vi "Main.vi"() -> ()   [LabVIEW 2016]
uses:
  Globale Variable/Globale Variable.vi
panel:
  in  "LAUNCH":bool
  in  "voltage_start":dbl
  in  "starting threshold":dbl
  in  "v_max":dbl
  in  "k_lqr":dbl
  out "error out":errorcluster
  in  "lambda_target":dbl=0.1
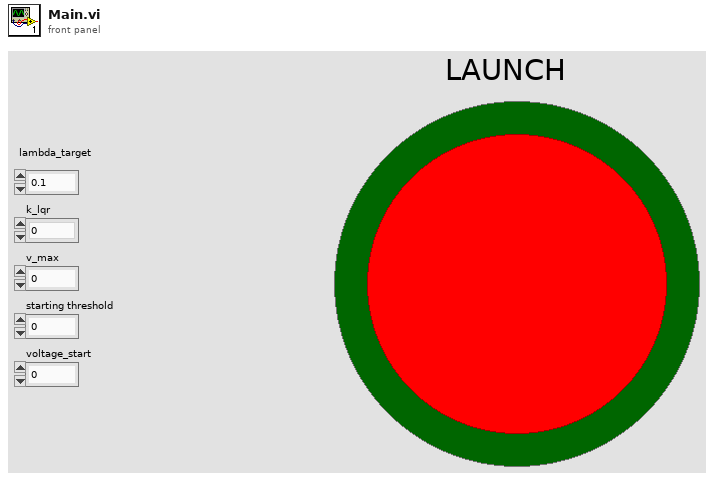
[diagram p1: front panel]
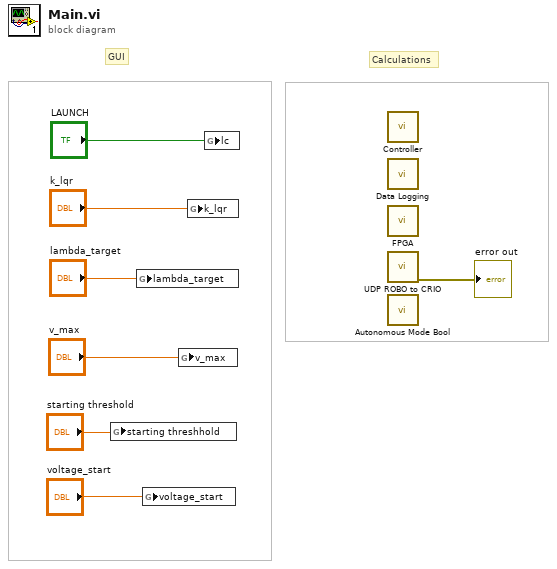
[diagram p0: block diagram]
diagram:
  # "Calculations"
  # "GUI"
  n1 = global write "Globale Variable.vi" "starting threshhold"("starting threshold") -> ()
  n2 = global write "Globale Variable.vi" "lambda_target"("lambda_target") -> ()
  n3 = global write "Globale Variable.vi" "voltage_start"("voltage_start") -> ()
  n4 = global write "Globale Variable.vi" "v_max"("v_max") -> ()
  n5 = global write "Globale Variable.vi" "k_lqr"("k_lqr") -> ()
  n6 = global write "Globale Variable.vi" "lc"("LAUNCH") -> ()
  n7 = call "Controller.vi"() -> ()  [unwired: 12 in]
  n8 = call "Data Logging.vi"() -> ()  [unwired: 12 in]
  n9 = call "FPGA.vi"() -> ()  [unwired: 12 in]
  n10 = call "UDP ROBO to CRIO.vi"() -> ("error out"=→"error out":errorcluster)  [unwired: 11 in]
  n11 = call "Autonomous Mode Bool.vi"() -> ()  [unwired: 12 in]
